vi "Convert Rectangle to Polygon.vi"(8 "error in (no error)":errorcluster, 11 "Rectangle":T2 {"Rotation" min=-90.0 max=90.0 step=1.0 format="%.2f"; "Left" scale=0.0..1024.0; "Right" scale=0.0..1024.0}) -> (0 "error out":errorcluster, 2 "Rotation":dbl, 3 "Rectangle Points":T1[](array[typedef]) {"Y" format="%.2f"; "X" format="%.2f"})   [LabVIEW 2015]
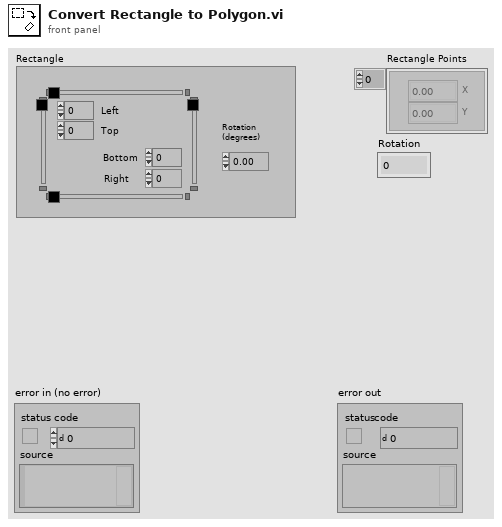
[diagram p1: front panel]
types:
  T1 = typedef "IMAQ Point" = cluster{"X":sgl, "Y":sgl}
  T2 = typedef "IMAQ Rectangle" = cluster{"Left":i32, "Top":i32, "Right":i32, "Bottom":i32, "Rotation":dbl}
  T3 = cluster{"Left":dbl, "Top":dbl, "Right":dbl, "Bottom":dbl, "Rotation":dbl}
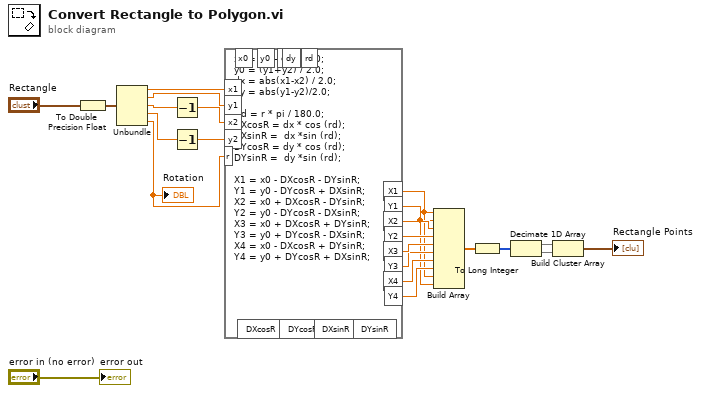
[diagram p0: block diagram]
diagram:
  n1 = To Double Precision Float(number="Rectangle") -> (double precision float=w18:T3)
  n2 = Unbundle(w18) -> ("Left"=w19:dbl, "Top"=w20:dbl, "Right"=w21:dbl, "Bottom"=w22:dbl, "Rotation"=w23:dbl)
  "Rotation" <- w23
  n3 = Decrement(x=w21) -> (x-1=w3:dbl)
  n4 = Decrement(x=w22) -> (x-1=w2:dbl)
  n5 = formula code="x0 = (x1+x2) / 2.0;\ny0 = (y1+y2) / 2.0;\ndx = abs(x1-x2) / 2.0;\ndy = abs(y1-y2)/2.0;\n\n rd = r * pi / 180.0;\nDXcosR = dx * cos (rd);\nDXsinR =  dx *sin (rd);\nDYcosR = dy * cos (rd);\nDYsinR =  dy *sin (rd);\n\nX1 = x0 - DXcosR - DYsinR;\nY1 = y0 - DYcosR + DXsinR;\nX2 = x0 + DXcosR - DYsinR;\nY2 = y0 - DYcosR - DXsinR;\nX3 = x0 + DXcosR + DYsinR;\nY3 = y0 + DYcosR - DXsinR;\nX4 = x0 - DXcosR + DYsinR;\nY4 = y0 + DYcosR + DXsinR;"("x2"=w3, "y2"=w2, "r"=w23, "x1"=w19, "y1"=w20) -> ("X1"=w6:dbl, "Y1"=w5:dbl, "X2"=w16:dbl, "Y2"=w15:dbl, "X3"=w14:dbl, "Y3"=w13:dbl, "X4"=w12:dbl, "Y4"=w11:dbl)  [unwired: 9 out]
  n6 = Build Array(w6, w5, w16, w15, w14, w13, w12, w11, w6, w5) -> (w10:dbl[])
  n7 = To Long Integer(number=w10) -> (32bit integer=w9:i32[])
  n8 = Decimate 1D Array(w9) -> (w7:i32[], w8:i32[])
  n9 = Build Cluster Array(w7, w8) -> (→"Rectangle Points":cluster{"Y1":i32, "Y1":i32}[])
  "error out" <- "error in (no error)"
